vi "Results.vi"(8 "error in (no error)":errorcluster, 11 "FFT in":refnum<class "FFT.lvclass">) -> (0 "error out":errorcluster, 3 "FFT out":refnum<class "FFT.lvclass">)   [LabVIEW 2018, in "AnalysisPlugins.lvlib" / "FFT.lvclass"]
uses:
  FFT.lvclass
  X:/Projects/PMUCal/Modules/Analysis/AnalysisPlugins/AnalysisPluginBaseClass/AnalysisPluginsBase.lvclass
  X:/Projects/PMUCal/Modules/Analysis/AnalysisPlugins/FitterBaseClass/FitterBase.lvclass
  Typedefs/FftReport.ctl
  AnalysisPluginBaseClass/AnalysisPluginsBase.lvclass/AnalysisPluginsBase.ctl
  AnalysisPluginBaseClass/Accessors/Read ResultPath.vi
  AnalysisPluginBaseClass/Accessors/Read Result.vi
  AnalysisPluginBaseClass/Accessors/Read Window.vi
  <vilib>/Analysis/Matrix/Numeric/Conversions/Matrix To Array - CM.vi
  <vilib>/Utility/file.llb/Write Delimited Spreadsheet (DBL).vi
  <vilib>/Analysis/Matrix/NI_Matrix.lvlib
panel:
  out "file name":string
  out "bin":dbl[](array[numeric])
  out "DFT bin Im":dbl
  out "DFT bin Re":dbl
  out "phase [rad]":dbl
  out "module [V]":dbl
  out "T0":timestamp
  out "TimeStamp":timestamp
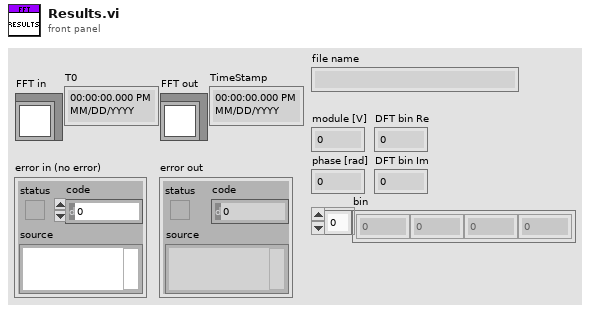
[diagram p1: front panel]
types:
  T1 = typedef "AnalysisPlugins.lvlib/FFT.lvclass/FftReport.ctl" = cluster{"dF":dbl, "FFT":cdb[][], "F0":dbl}
  T2 = typedef "AnalysisPlugins.lvlib/AnalysisPluginsBase.lvclass/clWindowData.ctl" = cluster{"Timestamp":ext, "Samples":dbl[][], "Window Valid":bool, "T0":ext}
  T3 = typedef "AnalysisPlugins.lvlib/FitterBase.lvclass/clAnalysisConfig.ctl" = cluster{"F0":u32, "SettlingTime":dbl, "AnalysisCycles":dbl, "SampleRate":dbl, "NumChannels":u32, "TsOffset":enum16{"start", "middle", "end"}}
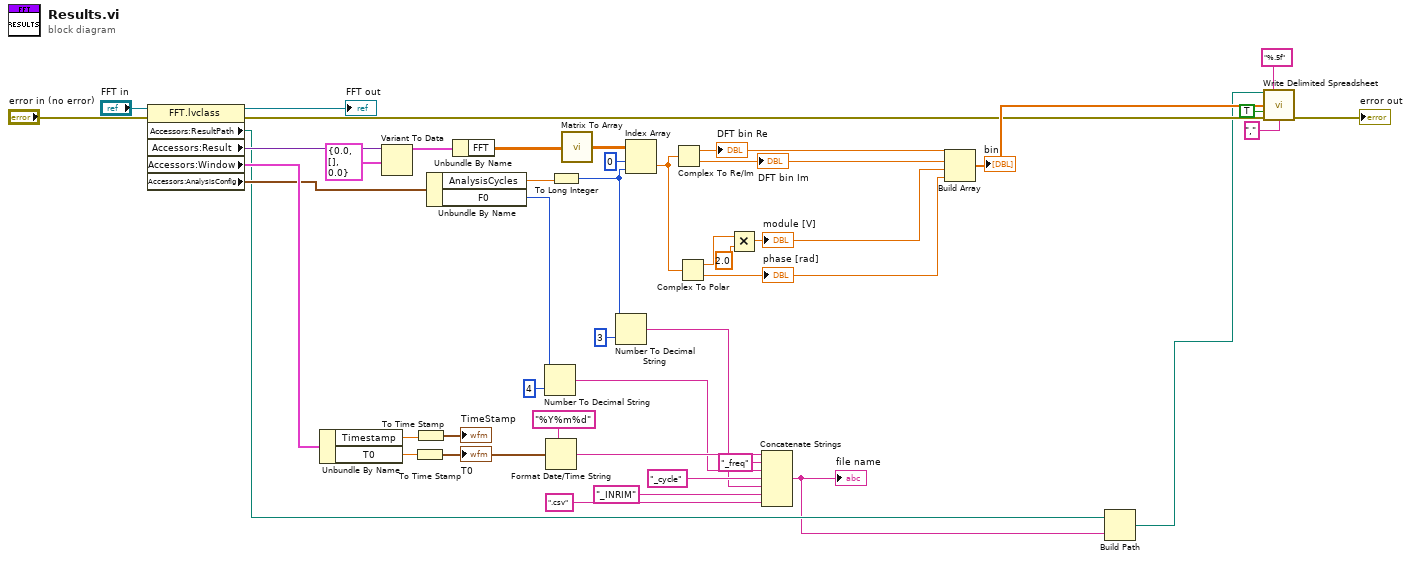
[diagram p0: block diagram]
diagram:
  n1 = property class="FFT.lvclass"(reference="FFT in", error in="error in (no error)") -> (reference out=→"FFT out":refnum<class "FFT.lvclass">, error out=w10:errorcluster, "Accessors:ResultPath"=w23:path, "Accessors:Result"=w42:variant, "Accessors:Window"=w40:T2, "Accessors:AnalysisConfig"=w35:T3)
  n2 = Unbundle By Name(w40) -> ("Timestamp"=w39:ext, "T0"=w38:ext)
  n3 = Variant To Data(type=T1 {"dF"=0.0, "FFT"=[], "F0"=0.0} ("FftReport"), Variant=w42) -> (data=w34:T1)  [unwired: 1 in, 1 out]
  n4 = To Time Stamp(1:w38) -> (0:w22:timestamp)
  "T0" <- w22
  n5 = To Time Stamp(1:w39) -> (0:→"TimeStamp":timestamp)
  n6 = Unbundle By Name(w35) -> ("AnalysisCycles"=w6:dbl, "F0"=w7:u32)
  n7 = Unbundle By Name(w34) -> ("FFT"=w33:cdb[][])
  n8 = Number To Decimal String(number=w7, width (-)=i16 4) -> (decimal integer string=w18:string)
  n9 = Format Date/Time String(time format string (%c)="%Y%m%d", seconds (now)=w22) -> (date/time string=w20:string)  [unwired: 1 in]
  n10 = To Long Integer(number=w6) -> (32bit integer=w5:i32)
  n11 = call-poly <vilib>:"Matrix To Array.vi"("Complex Matrix"=w33) -> ("Complex 2D Array"=w32:cdb[][])
  n12 = Number To Decimal String(number=w5, width (-)=i16 3) -> (decimal integer string=w16:string)
  n13 = Index Array(array=w32, index (row)=0, index (col)=w5) -> (element=w28:cdb)
  n14 = Complex To Re/Im(x + iy=w28) -> (x=w27:dbl, y=w26:dbl)
  "DFT bin Re" <- w27
  "DFT bin Im" <- w26
  n15 = Complex To Polar(r * e^(i*theta)=w28) -> (r=w30:dbl, theta=w24:dbl)
  "phase [rad]" <- w24
  n16 = Multiply(x=w30, y=2.0) -> (x*y=w25:dbl)
  "module [V]" <- w25
  n17 = Concatenate Strings(w20, "_freq" ("string"), w18, "_cycle" ("string"), w16, "_INRIM" ("string"), ".csv" ("string")) -> (w12:string)
  "file name" <- w12
  n18 = Build Array(w27, w26, w25, w24) -> (w11:dbl[])
  "bin" <- w11
  n19 = Build Path(base path=w23, name or relative path=w12) -> (appended path=w2:path)
  n20 = call-poly <vilib>:"Write Delimited Spreadsheet.vi"("file path (dialog if empty)"=w2, "format (%.3f)"="%.5f", "1D data"=w11, "append to file? (new file:F)"=TRUE, "error in (no error)"=w10, "delimiter (\\t)"="," ("delimiter (\\t)")) -> ("error out"=→"error out":errorcluster)  [unwired: 8 in, 1 out]
